vi "Ctor.vi"(4 "Timeout ms":i32, 8 "error in (no error)":errorcluster, 10 "Client Command Queue":T1, 11 "TCP Connection":refnum<k5>) -> (0 "error out":errorcluster, 3 "TCP Stream out":refnum<class "TCP Stream.lvclass">)   [LabVIEW 2020, in "Stream-TCP.lvlib" / "TCP Stream.lvclass"]
uses:
  TCP Stream.lvclass
  Client Command.ctl
  Stream-TCP.lvlib
  Client Command Queue.ctl
  Ref Data.ctl
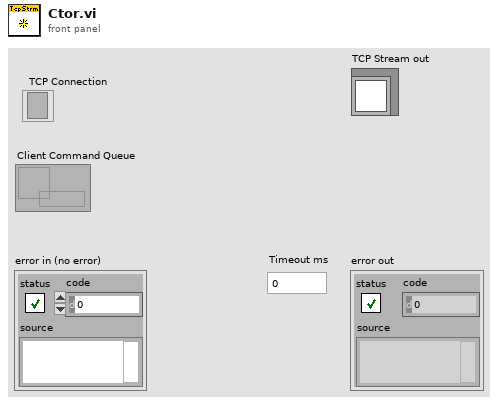
[diagram p1: front panel]
types:
  T1 = typedef "Stream-TCP.lvlib/Client Command Queue.ctl" = refnum<queue>
  T2 = typedef "Stream-TCP.lvlib/TCP Stream.lvclass/Ref Data.ctl" = cluster{"Client Command Queue":T1}
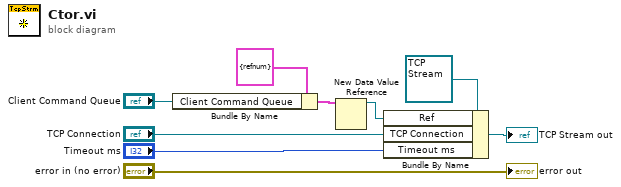
[diagram p0: block diagram]
diagram:
  n1 = Bundle By Name(cluster=T2 {"Client Command Queue"=refnum} ("Ref Data"), "Client Command Queue"="Client Command Queue") -> (w4:T2)
  n2 = New Data Value Reference(data value=w4) -> (data value reference=w2:refnum<data-value>)  [unwired: 1 in, 1 out]
  n3 = Bundle By Name(cluster=refnum<class "TCP Stream.lvclass"> refnum ("TCP Stream in"), "Ref"=w2, "TCP Connection"="TCP Connection", "Timeout ms"="Timeout ms") -> (→"TCP Stream out":refnum<class "TCP Stream.lvclass">)
  "error out" <- "error in (no error)"
